vi "Read Dev Rolloff.vi"(8 "error in (no error)":errorcluster, 11 "VISA resource name":refnum<visa-resource-name>) -> (0 "error out":errorcluster, 2 "dev rollofff":T1, 3 "VISA resource name out":refnum<visa-resource-name>)   [LabVIEW 2020, in "Andeen-Hagerling 2700A.lvlib"]
doc: "Returns the 3 db down point of the analog output frequency roll\noff limit. Both the setting and the actual rolloff are returned."
uses:
  Andeen-Hagerling 2700A.lvlib
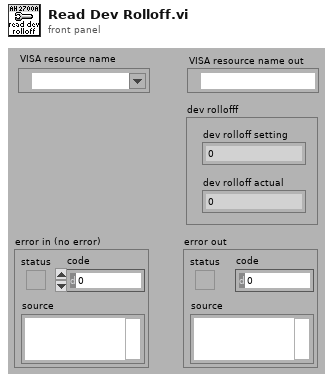
[diagram p1: front panel]
types:
  T1 = cluster{"dev rolloff setting":dbl, "dev rolloff actual":dbl}
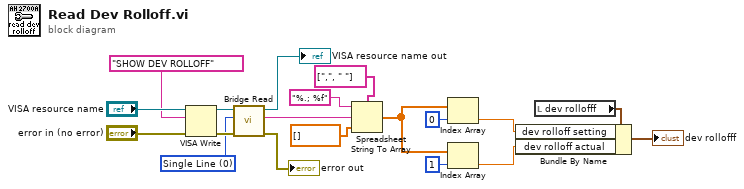
[diagram p0: block diagram]
diagram:
  w1 = u16 0 items=["Single Line", "Multi-Line"] ("Multiline")
  n1 = VISA Write(VISA resource name="VISA resource name", write buffer="SHOW DEV ROLLOFF" ("command"), error in (no error)="error in (no error)") -> (VISA resource name out=w6:refnum<visa-resource-name>, error out=w5:errorcluster)  [unwired: 1 out]
  n2 = call "Bridge Read.vi"("error in (no error)"=w5, "multiline"=w1, "VISA resource name"=w6) -> ("error out"=→"error out":errorcluster, "read buffer"=w3:string, "VISA resource name out"=→"VISA resource name out":refnum<visa-resource-name>)  [unwired: 6 in]
  n3 = Spreadsheet String To Array(delimiter (Tab)=string[] [",", " "], format string="%.; %f", spreadsheet string=w3, array type (2D Dbl)=dbl[] []) -> (array=w12:dbl[])
  n4 = Index Array(array=w12, index=0) -> (element=w9:dbl)
  n5 = Index Array(array=w12, index=1) -> (element=w8:dbl)
  n6 = local read "dev rollofff"() -> (w10:T1)
  n7 = Bundle By Name(cluster=w10, "dev rolloff setting"=w9, "dev rolloff actual"=w8) -> (→"dev rollofff":T1)
